vi "error function.vi"(3 "output control":T1, 4 "data":variant, 5 "X":dbl[](array[numeric]), 6 "a":dbl[](array[numeric])) -> (0 "error out":errorcluster, 1 "f'(X,a)":dbl[][](array[numeric]), 2 "f(X,a)":dbl[](array[numeric]))   [LabVIEW 2012]
uses:
  <vilib>/gmath/NumericalOptimization/LM_output select.ctl
  <vilib>/gmath/NI_Gmath.lvlib
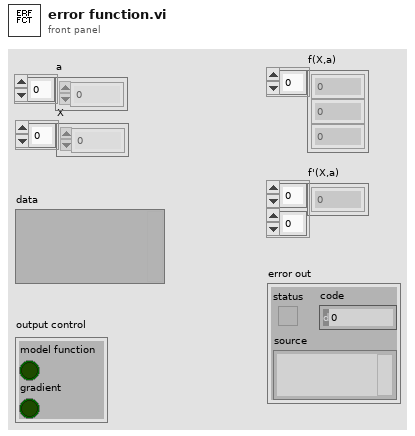
[diagram p1: front panel]
types:
  T1 = typedef "NI_Gmath.lvlib/LM_output select.ctl" = cluster{"model function":bool, "gradient":bool}
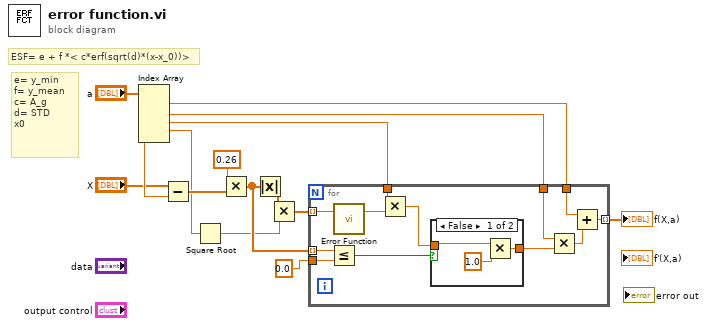
[diagram p0: block diagram]
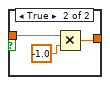
[diagram p2: hidden frame]
diagram:
  # "e= y_min\nf= y_mean\nc= A_g\nd= STD\nx0"
  # "ESF= e + f *< c*erf(sqrt(d)*(x-x_0))>"
  n1 = Index Array(array="a") -> (element #1=w14:dbl, element #2=w13:dbl, element #3=w12:dbl, element #4=w5:dbl, element #5=w9:dbl)  [unwired: 5 in]
  n2 = Subtract(x="X", y=w9) -> (x-y=w6:dbl[])
  n3 = Square Root(x=w5) -> (sqrt(x)=w3:dbl)
  n4 = Multiply(x=0.26, y=w6) -> (x*y=w10:dbl[])
  n5 = Absolute Value(x=w10) -> (abs(x)=w8:dbl[])
  n6 = Multiply(x=w8, y=w3) -> (x*y=w4:dbl[])
  n7 = for {
    tunnel: w4 -> [w27] mode=indexing
    tunnel: w10 -> [w26] mode=indexing
    tunnel: 0.0 -> [w25]
    tunnel: w12 -> [w23]
    tunnel: [w16] -> w15 mode=indexing
    tunnel: w13 -> [w18]
    tunnel: w14 -> [w17]
    n8 = Less Or Equal?(x=w26, y=w25) -> (x <= y?=w22:bool)
    n9 = call <vilib>:"Error Function.vi"("x"=w27) -> ("erf(x)"=w24:dbl)  [unwired: 2 in]
    n10 = Multiply(x=w23, y=w24) -> (x*y=w21:dbl)
    n11 = case shown="False" w22 {
      tunnel: w21 -> [w29 w32]
      tunnel: [w28 w31] -> w19
      frame False {
        n12 = Multiply(x=w29, y=1.0) -> (x*y=w28:dbl)
      }
      frame True {
        n13 = Multiply(x=w32, y=-1.0) -> (x*y=w31:dbl)
      }
    }
    n14 = Multiply(x=w18, y=w19) -> (x*y=w20:dbl)
    n15 = Add(x=w17, y=w20) -> (x+y=w16:dbl)
  }
  "f(X,a)" <- w15
